vi "Set Hardware Relay State.vi"(0 "RelayInterface in":refnum<class "RelayInterface.lvclass">, 5 "session in":refnum<k21>, 7 "device in":refnum<k21>, 9 "relay action (Close Relay)":T1=1 items=["Open Relay", "Close Relay"], 11 "error in (no error)":errorcluster) -> (4 "RelayInterface out":refnum<class "RelayInterface.lvclass">, 6 "session out":refnum<k21>, 8 "device out":refnum<k21>, 15 "error out":errorcluster)   [LabVIEW 2015, in "RelayInterface.lvclass"]
uses:
  RelayInterface.lvclass
  slscsl/RelayAction.ctl
  slscsl/slscsl.lvclass
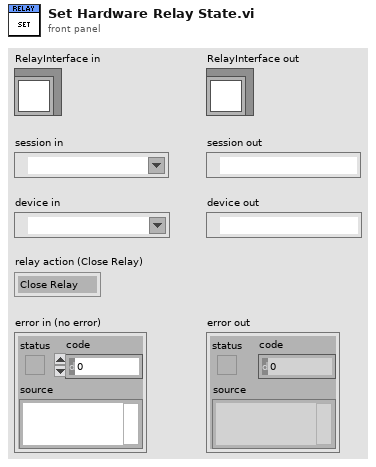
[diagram p1: front panel]
types:
  T1 = typedef "slscsl.lvclass/RelayAction.ctl" = u16
  T2 = typedef "slscsl.lvclass/RelayPosition.ctl" = i32
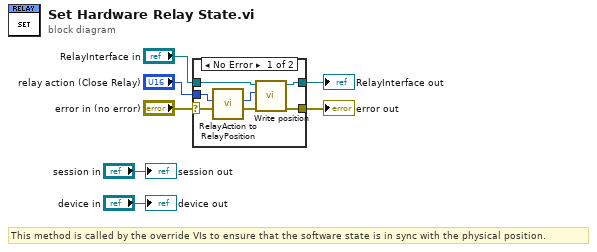
[diagram p0: block diagram]
diagram:
  # "This method is called by the override VIs to ensure that the software state is in sync with the physical position."
  n1 = case shown="No Error" "error in (no error)" {
    selector: "error in (no error)" -> [w9 w15]
    tunnel: [w8 w15] -> w6
    tunnel: [w12 w14] -> w4
    tunnel: "RelayInterface in" -> [w13 w14]
    tunnel: "relay action (Close Relay)" -> [w11 _]
    frame No Error {
      n2 = call "RelayAction to RelayPosition.vi"("action"=w11) -> ("position"=w10:T2)  [unwired: 10 in]
      n3 = call-dynamic "Write position.vi"("error in (no error)"=w9, "position"=w10, "RelayInterface in"=w13) -> ("error out"=w8:errorcluster, "RelayInterface out"=w12:refnum<class "RelayInterface.lvclass">)  [unwired: 7 in]
    }
    frame Error {
    }
  }
  "error out" <- w6
  "RelayInterface out" <- w4
  "device out" <- "device in"
  "session out" <- "session in"
